vi "加标仪器启动命令 (子VI).vi"(8 "错误输入（无错误）":errorcluster, 10 "启动命令":enum16{"启动水样流程", "启动加标流程", "排液", "停止", "柱塞泵启动"}(ring), 11 "仪器":enum16{"", "氨氮", "总磷", "总氮", "CODMn", "CODCr"}(ring)=enum."氨氮") -> (0 "错误输出":errorcluster)   [LabVIEW 2016, in "质控单元.lvlib"]
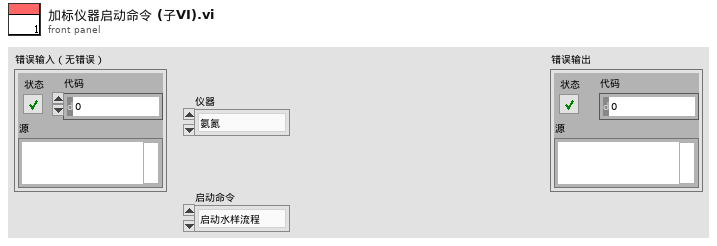
[diagram p1: front panel]
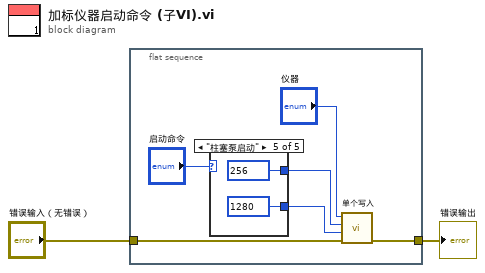
[diagram p0: block diagram]
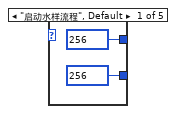
[diagram p2: hidden frame]
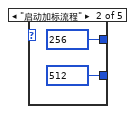
[diagram p3: hidden frame]
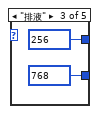
[diagram p4: hidden frame]
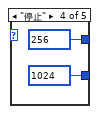
[diagram p5: hidden frame]
diagram:
  n1 = flat-sequence {
    tunnel: [w3] -> w1
    tunnel: "错误输入（无错误）" -> [w4]
    frame #0 {
      n2 = case shown="\"柱塞泵启动\"" "启动命令" {
        tunnel: [u16 256 ("starting address") u16 256 ("starting address") u16 256 ("starting address") u16 256 ("starting address") u16 256 ("starting address")] -> w6
        tunnel: [u16 256 ("starting address") u16 512 ("starting address") u16 768 ("starting address") u16 1024 ("starting address") u16 1280 ("starting address")] -> w5
        frame "启动水样流程", Default {
        }
        frame "启动加标流程" {
        }
        frame "排液" {
        }
        frame "停止" {
        }
        frame "柱塞泵启动" {
        }
      }
      n3 = call "单个写入.vi"("Error in"=w4, "value"=w5, "address"=w6, "Slave ID"="仪器") -> ("error out"=w3:errorcluster)  [unwired: 7 in]
    }
  }
  "错误输出" <- w1
